vi "ADC_BinFreq_Compare.vi"(1 "Fsample":dbl, 2 "# of Samples":i32, 5 "Expected Frequency":dbl format="%#_13g", 11 "error in":errorcluster, 12 "Input Freq":dbl format="%#_8g", 13 "+/- error(bins)":i32, 14 "F units":u16(ring) items=["Hz", "KHz", "MHz"]) -> (3 "In Range?(T)":bool, 4 "bin":dbl format="%#_8f", 6 "lsl/hsl/bin":dbl[](array[numeric]), 15 "error out":errorcluster)   [LabVIEW 2018]
panel:
  out "time":dbl
  in  "Export Table to Excel":bool
  out "BinFreqs":dbl[](array[numeric]) format="%#_8g"
  out "subarray":dbl[](array[numeric])
  out "closest element":dbl
  out "lower limit":dbl
  out "upper limit":dbl
  out "Numeric":dbl
  # "Generate the Sample Table"
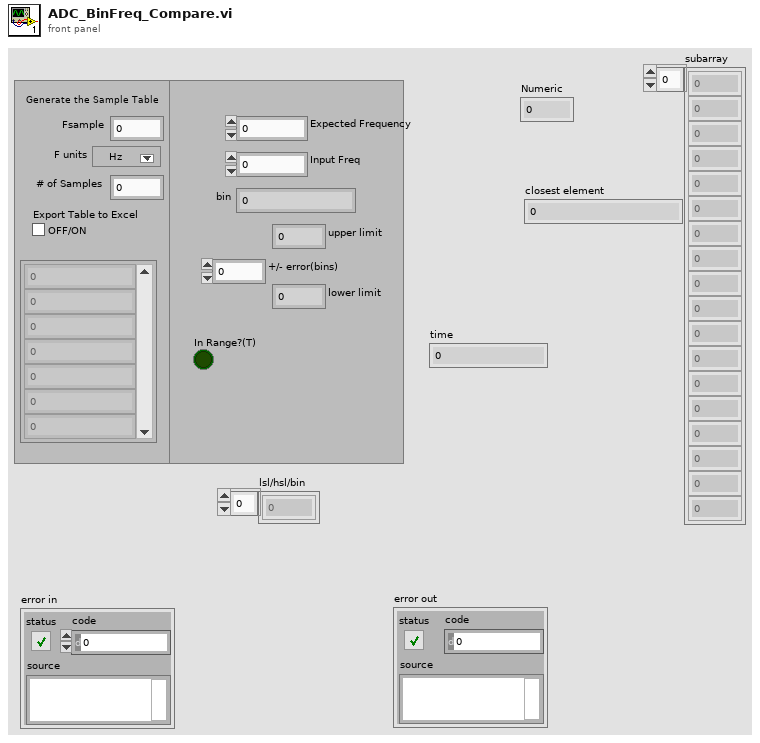
[diagram p1: front panel]
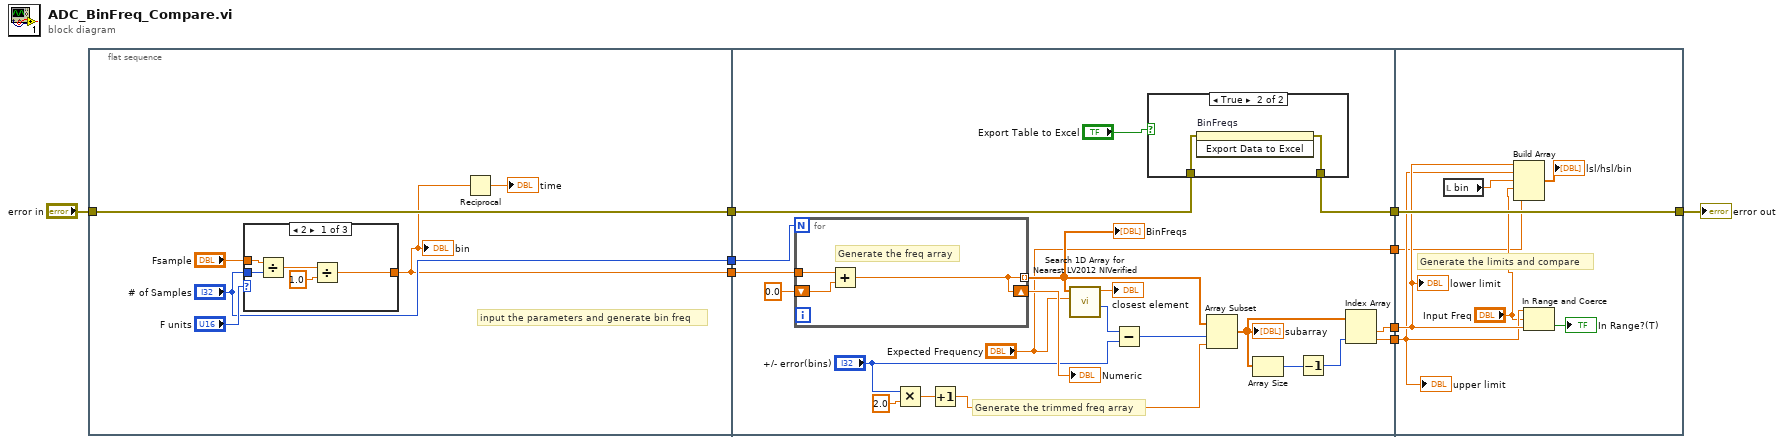
[diagram p0: block diagram]
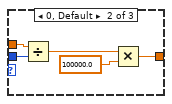
[diagram p2: hidden frame]
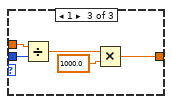
[diagram p3: hidden frame]
diagram:
  n1 = flat-sequence {
    tunnel: ["# of Samples"] -> w9
    tunnel: [w11] -> w8
    tunnel: "error in" -> [w12]
    tunnel: [w12] -> w4
    tunnel: w9 -> [w50]
    tunnel: w8 -> [w49]
    tunnel: [w38] -> w7
    tunnel: [w37] -> w6
    tunnel: w4 -> [w34]
    tunnel: [w33] -> w3
    tunnel: ["Expected Frequency"] -> w1
    tunnel: w7 -> [w63]
    tunnel: w6 -> [w62]
    tunnel: w3 -> [w64]
    tunnel: [w64] -> w2
    tunnel: w1 -> [w58]
    frame #0 {
      # "input the parameters and generate bin freq"
      n2 = case shown="2" "F units" {
        tunnel: "Fsample" -> [w19 w24 w29]
        tunnel: [w17 w22 w27] -> w11
        tunnel: "# of Samples" -> [w20 w25 w30]
        frame 2 {
          n3 = Divide(x=w19, y=w20) -> (x/y=w18:dbl)
          n4 = Divide(x=w18, y=1.0 ("x")) -> (x/y=w17:dbl)
        }
        frame 0, Default {
          n5 = Divide(x=w24, y=w25) -> (x/y=w23:dbl)
          n6 = Multiply(x=w23, y=100000.0 ("x")) -> (x*y=w22:dbl)
        }
        frame 1 {
          n7 = Divide(x=w29, y=w30) -> (x/y=w28:dbl)
          n8 = Multiply(x=w28, y=1000.0 ("x")) -> (x*y=w27:dbl)
        }
      }
      "bin" <- w11
      n9 = Reciprocal(x=w11) -> (1/x=→"time":dbl)
    }
    frame #1 {
      # "Generate the trimmed freq array"
      n10 = for {
        N: w50 -> [_]
        tunnel: w49 -> [w57]
        shift-right: [w55] -> w51
        shift-left: 0.0 -> [w56]
        tunnel: [w55] -> w46 mode=indexing
        # "Generate the freq array"
        n11 = Add(x=w57, y=w56) -> (x+y=w55:dbl)
      }
      "BinFreqs" <- w46
      "Numeric" <- w51
      n12 = Multiply(x="+/- error(bins)", y=2.0) -> (x*y=w44:dbl)
      n13 = Increment(x=w44) -> (x+1=w41:dbl)
      n14 = call "Search 1D Array for Nearest LV2012 NIVerified.vi"("desired element"="Expected Frequency", "1D Array"=w46) -> ("closest index"=w43:i32, "closest element"=→"closest element":dbl)  [unwired: 8 in]
      n15 = Subtract(x=w43, y="+/- error(bins)") -> (x-y=w45:i32)
      n16 = case shown="True" "Export Table to Excel" {
        tunnel: w34 -> [w52 w54]
        tunnel: [w52 w53] -> w33
        frame False {
        }
        frame True {
          n17 = invoke on="BinFreqs" class="Arr (strict)" method="Export Data to Excel"(error in=w54) -> (error out=w53:errorcluster)  [unwired: 2 in, 2 out]
        }
      }
      n18 = Array Subset(array=w46, index=w45, length=w41) -> (w39:dbl[])
      "subarray" <- w39
      n19 = Array Size(array=w39) -> (size(s)=w40:i32)
      n20 = Decrement(x=w40) -> (x-1=w36:i32)
      n21 = Index Array(array=w39, index #2=w36) -> (element #1=w38:dbl, element #2=w37:dbl)  [unwired: 1 in]
    }
    frame #2 {
      # "Generate the limits and compare"
      n22 = local read "bin"() -> (w60:dbl)
      n23 = Build Array(w63, w62, w60, "Input Freq", w58) -> (→"lsl/hsl/bin":dbl[])
      n24 = In Range and Coerce(upper limit=w62, x="Input Freq", lower limit=w63) -> (In Range?=→"In Range?(T)":bool)  [unwired: 1 out]
      "upper limit" <- w62
      "lower limit" <- w63
    }
  }
  "error out" <- w2
